vi "Write Text.vi"(8 "error in (no error)":errorcluster, 9 "Text":string, 11 "Character LCD in":refnum<class "Grove I2C LCD.lvclass">) -> (0 "error out":errorcluster, 3 "Character LCD out":refnum<class "Grove I2C LCD.lvclass">)   [LabVIEW 2020, in "CTI-Peripheral.lvlib" / "Grove I2C LCD.lvclass"]
uses:
  Grove I2C LCD.lvclass
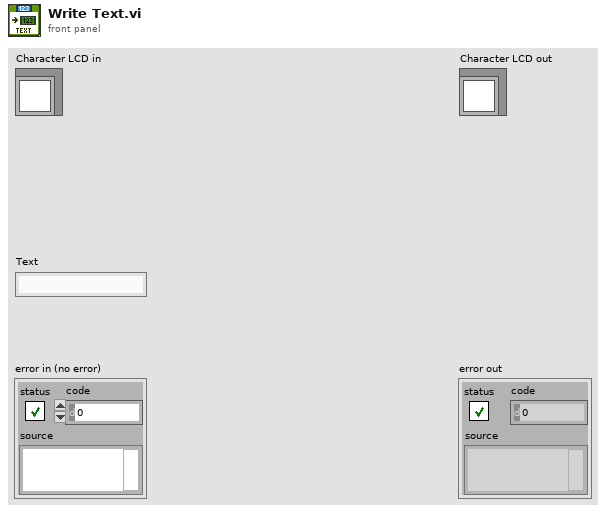
[diagram p1: front panel]
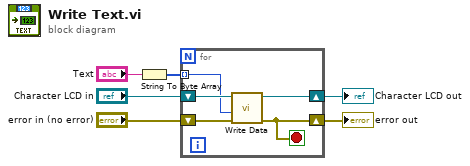
[diagram p0: block diagram]
diagram:
  n1 = String To Byte Array(string="Text") -> (unsigned byte array=w1:u8[])
  n2 = for {
    shift-right: [w7] -> w4
    shift-left: "error in (no error)" -> [w11]
    shift-right: [w9] -> w2
    shift-left: "Character LCD in" -> [w10]
    tunnel: w1 -> [w8] mode=indexing
    stop <- w7 stop-if-true
    n3 = call "Write Data.vi"("error in (no error)"=w11, "Value"=w8, "Grove I2C LCD in"=w10) -> ("error out"=w7:errorcluster, "Grove I2C LCD out"=w9:refnum<class "Grove I2C LCD.lvclass">)  [unwired: 7 in]
  }
  "error out" <- w4
  "Character LCD out" <- w2
